vi "Test Serial 2.vi"() -> ()   [LabVIEW 2014]
uses:
  <vilib>/LabVIEW Universal Transcriptor/LabVIEW to Arduino Transcriptor/Transcriptors/System API/System Serial Library Variables/System Serial Library Variables.lvlib
panel:
  out "Error Out":errorcluster
  in  "Error In":errorcluster
  out "Serial Status":string
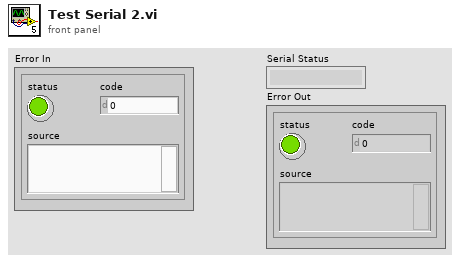
[diagram p1: front panel]
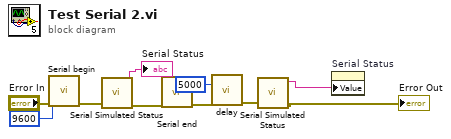
[diagram p0: block diagram]
diagram:
  n1 = call <vilib>:"Serial begin.vi"("Error In"="Error In", "speed (Bd)"=9600) -> ("Error Out"=w10:errorcluster)  [unwired: 9 in]
  n2 = call <vilib>:"Serial Simulated Status.vi"("error in (no error)"=w10) -> ("error out"=w9:errorcluster, "Serial Status"=→"Serial Status":string)  [unwired: 9 in]
  n3 = call <vilib>:"Serial end.vi"("Error In"=w9) -> ("Error Out"=w3:errorcluster)  [unwired: 10 in]
  n4 = call <vilib>:"delay.vi"("Error In"=w3, "time (ms)"=5000) -> ("Error Out"=w2:errorcluster)  [unwired: 9 in]
  n5 = call <vilib>:"Serial Simulated Status.vi"("error in (no error)"=w2) -> ("error out"=→"Error Out":errorcluster, "Serial Status"=w4:string)  [unwired: 9 in]
  n6 = property on="Serial Status" class="Str"("Value"=w4) -> ()  [unwired: 2 in, 2 out]
